vi "Set Pre Trigger Percent.vi"(8 "error in (no error)":errorcluster, 11 "front":i32) -> (0 "error out":errorcluster)   [LabVIEW 2021, in "vmmso.lvlib"]
doc: "DLL_API void WINAPI SetPreTriggerPercent(int front);"
uses:
  vmmso.lvlib
  vmmso.dll
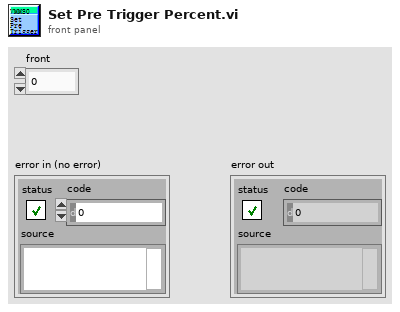
[diagram p1: front panel]
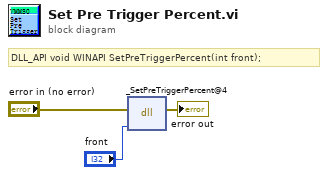
[diagram p0: block diagram]
diagram:
  # "DLL_API void WINAPI SetPreTriggerPercent(int front);"
  n1 = dll-call lib="O:/MSO/library/demo-Labview/vmmso/vmmso.*" fn="_SetPreTriggerPercent@4"(error in="error in (no error)", "front"="front") -> (error out=→"error out":errorcluster)  [unwired: 4 in, 1 out]
